vi "Send Enable Cancel.vi"(8 "error in (no error)":errorcluster, 11 "Build Events API in":refnum<class "Build Events API.lvclass">) -> (0 "error out":errorcluster, 3 "Build Events API out":refnum<class "Build Events API.lvclass">)   [LabVIEW 2020, in "Builder Tools.lvlib" / "Build Events API.lvclass"]
uses:
  Build Events API.lvclass
  Build Events API.lvclass/Build Events API.ctl
  Enable Cancel Data.ctl
  Builder Tools.lvlib
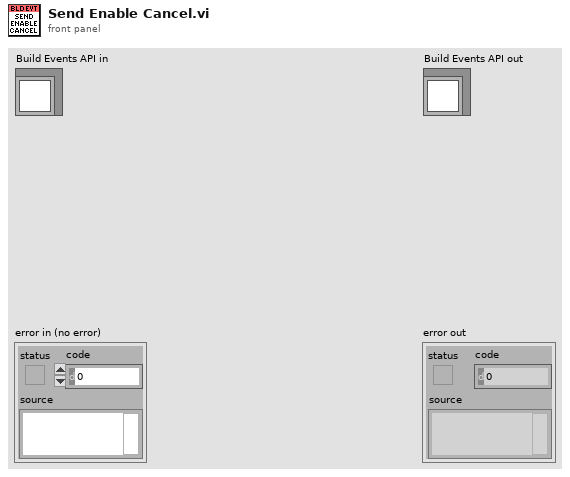
[diagram p1: front panel]
types:
  T1 = typedef "Builder Tools.lvlib/Enable Cancel Data.ctl" = cluster{"Unused":bool}
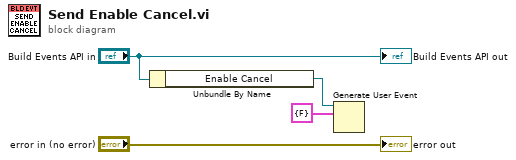
[diagram p0: block diagram]
diagram:
  n1 = Unbundle By Name("Build Events API in") -> ("Enable Cancel"=w2:refnum<user-event>)
  n2 = Generate User Event(user event=w2, event data cluster=T1 {"Unused"=FALSE} ("event data")) -> ()  [unwired: 2 in, 2 out]
  "error out" <- "error in (no error)"
  "Build Events API out" <- "Build Events API in"
